vi "hw5_2_(2) - test.vi"() -> ()   [LabVIEW 2014]
panel:
  out "Display":string
  in  "stop":bool
  out "Result":string
  in  "Calculator":T1
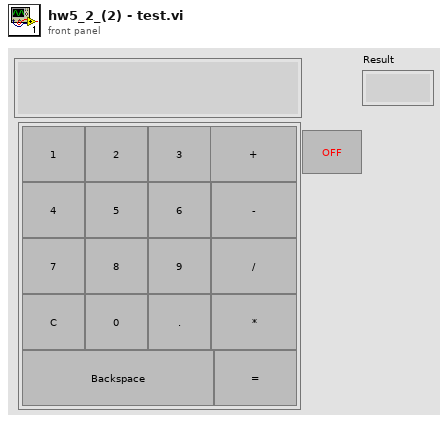
[diagram p1: front panel]
types:
  T1 = cluster{"2":bool, "3":bool, "4":bool, "5":bool, "6":bool, "7":bool, "8":bool, "9":bool, "*":bool, "=":bool, "backspace":bool, "0":bool, ".":bool, "C":bool, "/":bool, "-":bool, "+":bool, "1":bool}
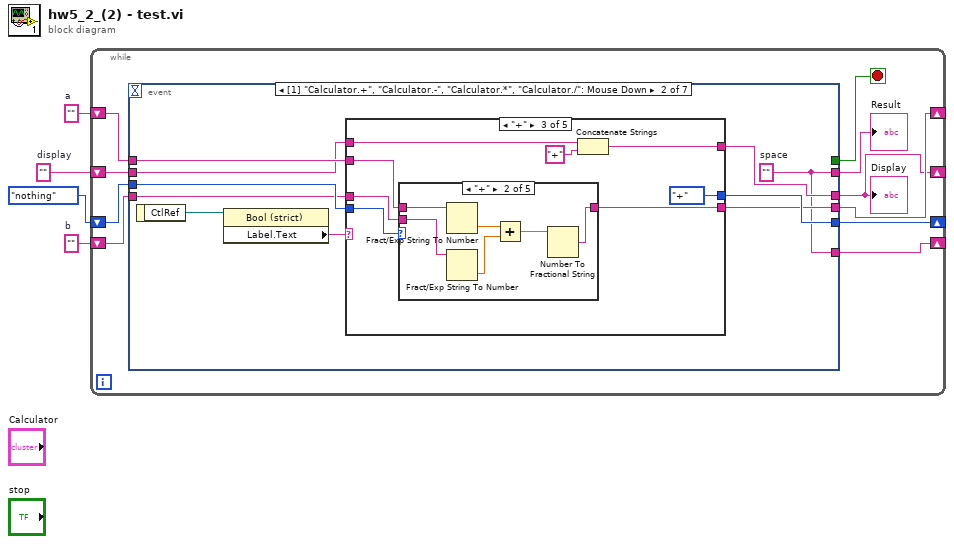
[diagram p0: block diagram]
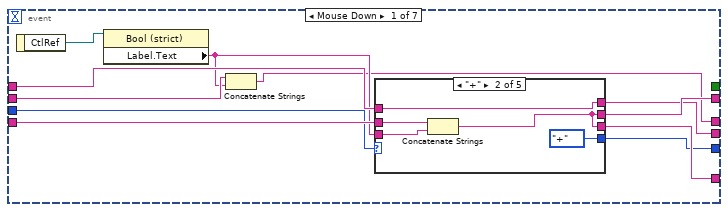
[diagram p2: hidden frame]
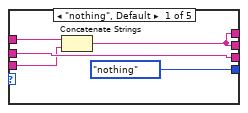
[diagram p3: hidden frame]
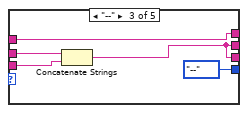
[diagram p4: hidden frame]
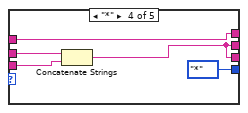
[diagram p5: hidden frame]
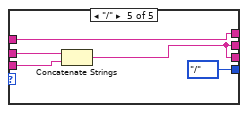
[diagram p6: hidden frame]
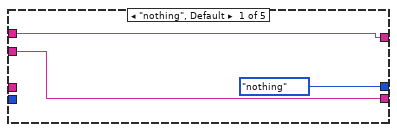
[diagram p7: hidden frame]
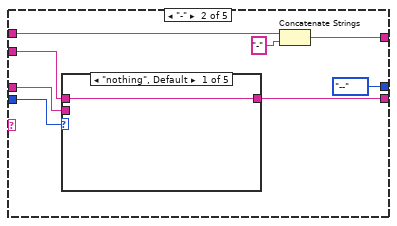
[diagram p8: hidden frame]
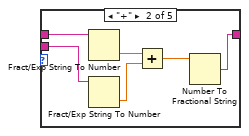
[diagram p9: hidden frame]
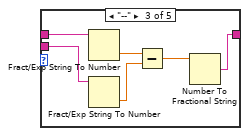
[diagram p10: hidden frame]
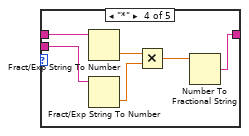
[diagram p11: hidden frame]
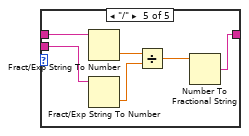
[diagram p12: hidden frame]
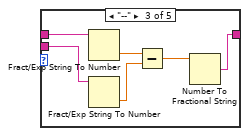
[diagram p14: hidden frame]
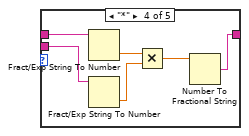
[diagram p15: hidden frame]
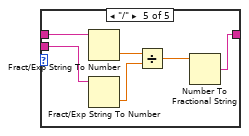
[diagram p16: hidden frame]
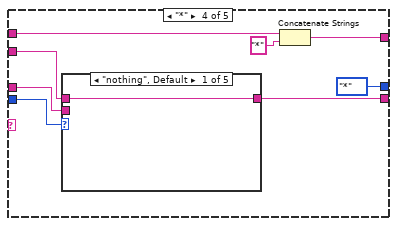
[diagram p17: hidden frame]
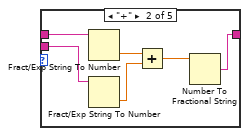
[diagram p18: hidden frame]
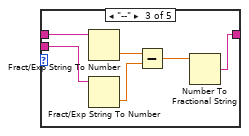
[diagram p19: hidden frame]
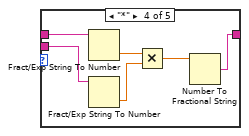
[diagram p20: hidden frame]
diagram:
  w1 = ""  # display
  w2 = ""  # b
  w4 = ""  # a
  n1 = while {
    shift-right: [w8] -> _
    shift-left: w4 -> [w14]
    shift-right: [w13] -> _
    shift-left: enum16{"nothing", "+", "--", "*", "/"}."nothing" -> [w10]
    shift-right: [w11] -> _
    shift-left: w2 -> [w12]
    shift-right: [w5] -> _
    shift-left: w1 -> [w6]
    stop <- w7 stop-if-true
    n2 = event shown="[1] \"Calculator.+\", \"Calculator.-\", \"Calculator.*\", \"Calculator./\": Mouse Down" {
      selector: _ -> [_ _ _ _ _ _ _]
      dyn-events: _ -> [_ _ _ _ _ _ _]
      timeout: _ -> [_ _ _ _ _ _ _]
      tunnel: w14 -> [w24 w58 w198 w241 w277 _ _]
      tunnel: [w18 w57 enum16{"nothing", "+", "--", "*", "/"}."nothing" w242 w281 _ _] -> w13
      tunnel: w12 -> [w23 w52 w197 w238 w276 _ _]
      tunnel: [w21 w51 w204 w243 w280 w312 _] -> w11
      tunnel: w10 -> [w19 w53 w199 w239 w275 _ _]
      tunnel: [w22 w51 w196 w244 w279 w312 _] -> w9
      tunnel: [w20 w56 w196 w245 w278 w312 _] -> w8
      tunnel: [_ _ _ _ _ _ TRUE] -> w7
      tunnel: w6 -> [w17 w54 w203 w237 w272 _ _]
      tunnel: [w15 w55 w200 w235 w271 w312 _] -> w5
      event "Calculator.1", "Calculator.2", "Calculator.3", "Calculator.4", "Calculator.5", "Calculator.6", "Calculator.7", "Calculator.8", "Calculator.9", "Calculator.0": Mouse Down {
        n3 = event-data() -> ("CtlRef"=w25:refnum<vi>)  [unwired: 1 in]
        n4 = property class="Bool (strict)"(reference=w25) -> ("Label.Text"=w16:string)  [unwired: 1 in, 2 out]
        n5 = Concatenate Strings(w17, w16) -> (w15:string)
        n6 = case shown="\"+\"" w19 {
          tunnel: w24 -> [w29 w34 w39 w44 w49]
          tunnel: w16 -> [w26 w31 w36 w41 w46]
          tunnel: [w27 w32 w37 w42 w48] -> w22
          tunnel: w23 -> [w30 w35 w40 w45 w50]
          tunnel: [w30 w32 w37 w42 w48] -> w21
          tunnel: [w27 w34 w39 w44 w49] -> w20
          tunnel: [enum16{"nothing", "+", "--", "*", "/"}."nothing" enum16{"nothing", "+", "--", "*", "/"}."+" enum16{"nothing", "+", "--", "*", "/"}."--" enum16{"nothing", "+", "--", "*", "/"}."*" enum16{"nothing", "+", "--", "*", "/"}."/"] -> w18
          frame "nothing", Default {
            n7 = Concatenate Strings(w29, w26) -> (w27:string)
          }
          frame "+" {
            n8 = Concatenate Strings(w35, w31) -> (w32:string)
          }
          frame "--" {
            n9 = Concatenate Strings(w40, w36) -> (w37:string)
          }
          frame "*" {
            n10 = Concatenate Strings(w45, w41) -> (w42:string)
          }
          frame "/" {
            n11 = Concatenate Strings(w50, w46) -> (w48:string)
          }
        }
      }
      event "Calculator.+", "Calculator.-", "Calculator.*", "Calculator./": Mouse Down {
        w51 = ""  # space
        n12 = event-data() -> ("CtlRef"=w60:refnum<vi>)  [unwired: 1 in]
        n13 = property class="Bool (strict)"(reference=w60) -> ("Label.Text"=w59:string)  [unwired: 1 in, 2 out]
        n14 = case shown="\"+\"" w59 {
          tunnel: w52 -> [_ w65 w98 w131 w164]
          tunnel: [w63 w67 w100 w133 w166] -> w56
          tunnel: w58 -> [w63 w71 w104 w137 w170]
          tunnel: [enum16{"nothing", "+", "--", "*", "/"}."nothing" enum16{"nothing", "+", "--", "*", "/"}."--" enum16{"nothing", "+", "--", "*", "/"}."+" enum16{"nothing", "+", "--", "*", "/"}."*" enum16{"nothing", "+", "--", "*", "/"}."/"] -> w57
          tunnel: [w61 w69 w102 w135 w168] -> w55
          tunnel: w54 -> [w61 w66 w99 w132 w165]
          tunnel: w53 -> [_ w64 w97 w130 w163]
          frame "nothing", Default {
          }
          frame "-" {
            n15 = case shown="\"nothing\", Default" w64 {
              tunnel: w71 -> [w72 w78 w84 w90 w96]
              tunnel: [w72 w77 w83 w89 w95] -> w67
              tunnel: w65 -> [_ w74 w80 w86 w92]
              frame "nothing", Default {
              }
              frame "+" {
                n16 = Fract/Exp String To Number(string=w78) -> (number=w75:dbl)  [unwired: 3 in, 1 out]
                n17 = Fract/Exp String To Number(string=w74) -> (number=w76:dbl)  [unwired: 3 in, 1 out]
                n18 = Add(x=w75, y=w76) -> (x+y=w73:dbl)
                n19 = Number To Fractional String(number=w73) -> (F-format string=w77:string)  [unwired: 3 in]
              }
              frame "--" {
                n20 = Fract/Exp String To Number(string=w84) -> (number=w81:dbl)  [unwired: 3 in, 1 out]
                n21 = Fract/Exp String To Number(string=w80) -> (number=w82:dbl)  [unwired: 3 in, 1 out]
                n22 = Subtract(x=w81, y=w82) -> (x-y=w79:dbl)
                n23 = Number To Fractional String(number=w79) -> (F-format string=w83:string)  [unwired: 3 in]
              }
              frame "*" {
                n24 = Fract/Exp String To Number(string=w90) -> (number=w87:dbl)  [unwired: 3 in, 1 out]
                n25 = Fract/Exp String To Number(string=w86) -> (number=w88:dbl)  [unwired: 3 in, 1 out]
                n26 = Multiply(x=w87, y=w88) -> (x*y=w85:dbl)
                n27 = Number To Fractional String(number=w85) -> (F-format string=w89:string)  [unwired: 3 in]
              }
              frame "/" {
                n28 = Fract/Exp String To Number(string=w96) -> (number=w93:dbl)  [unwired: 3 in, 1 out]
                n29 = Fract/Exp String To Number(string=w92) -> (number=w94:dbl)  [unwired: 3 in, 1 out]
                n30 = Divide(x=w93, y=w94) -> (x/y=w91:dbl)
                n31 = Number To Fractional String(number=w91) -> (F-format string=w95:string)  [unwired: 3 in]
              }
            }
            n32 = Concatenate Strings(w66, "-") -> (w69:string)
          }
          frame "+" {
            n33 = case shown="\"+\"" w97 {
              tunnel: w104 -> [w105 w111 w117 w123 w129]
              tunnel: [w105 w110 w116 w122 w128] -> w100
              tunnel: w98 -> [_ w107 w113 w119 w125]
              frame "nothing", Default {
              }
              frame "+" {
                n34 = Fract/Exp String To Number(string=w111) -> (number=w108:dbl)  [unwired: 3 in, 1 out]
                n35 = Fract/Exp String To Number(string=w107) -> (number=w109:dbl)  [unwired: 3 in, 1 out]
                n36 = Add(x=w108, y=w109) -> (x+y=w106:dbl)
                n37 = Number To Fractional String(number=w106) -> (F-format string=w110:string)  [unwired: 3 in]
              }
              frame "--" {
                n38 = Fract/Exp String To Number(string=w117) -> (number=w114:dbl)  [unwired: 3 in, 1 out]
                n39 = Fract/Exp String To Number(string=w113) -> (number=w115:dbl)  [unwired: 3 in, 1 out]
                n40 = Subtract(x=w114, y=w115) -> (x-y=w112:dbl)
                n41 = Number To Fractional String(number=w112) -> (F-format string=w116:string)  [unwired: 3 in]
              }
              frame "*" {
                n42 = Fract/Exp String To Number(string=w123) -> (number=w120:dbl)  [unwired: 3 in, 1 out]
                n43 = Fract/Exp String To Number(string=w119) -> (number=w121:dbl)  [unwired: 3 in, 1 out]
                n44 = Multiply(x=w120, y=w121) -> (x*y=w118:dbl)
                n45 = Number To Fractional String(number=w118) -> (F-format string=w122:string)  [unwired: 3 in]
              }
              frame "/" {
                n46 = Fract/Exp String To Number(string=w129) -> (number=w126:dbl)  [unwired: 3 in, 1 out]
                n47 = Fract/Exp String To Number(string=w125) -> (number=w127:dbl)  [unwired: 3 in, 1 out]
                n48 = Divide(x=w126, y=w127) -> (x/y=w124:dbl)
                n49 = Number To Fractional String(number=w124) -> (F-format string=w128:string)  [unwired: 3 in]
              }
            }
            n50 = Concatenate Strings(w99, "+") -> (w102:string)
          }
          frame "*" {
            n51 = case shown="\"nothing\", Default" w130 {
              tunnel: w137 -> [w138 w144 w150 w156 w162]
              tunnel: [w138 w143 w149 w155 w161] -> w133
              tunnel: w131 -> [_ w140 w146 w152 w158]
              frame "nothing", Default {
              }
              frame "+" {
                n52 = Fract/Exp String To Number(string=w144) -> (number=w141:dbl)  [unwired: 3 in, 1 out]
                n53 = Fract/Exp String To Number(string=w140) -> (number=w142:dbl)  [unwired: 3 in, 1 out]
                n54 = Add(x=w141, y=w142) -> (x+y=w139:dbl)
                n55 = Number To Fractional String(number=w139) -> (F-format string=w143:string)  [unwired: 3 in]
              }
              frame "--" {
                n56 = Fract/Exp String To Number(string=w150) -> (number=w147:dbl)  [unwired: 3 in, 1 out]
                n57 = Fract/Exp String To Number(string=w146) -> (number=w148:dbl)  [unwired: 3 in, 1 out]
                n58 = Subtract(x=w147, y=w148) -> (x-y=w145:dbl)
                n59 = Number To Fractional String(number=w145) -> (F-format string=w149:string)  [unwired: 3 in]
              }
              frame "*" {
                n60 = Fract/Exp String To Number(string=w156) -> (number=w153:dbl)  [unwired: 3 in, 1 out]
                n61 = Fract/Exp String To Number(string=w152) -> (number=w154:dbl)  [unwired: 3 in, 1 out]
                n62 = Multiply(x=w153, y=w154) -> (x*y=w151:dbl)
                n63 = Number To Fractional String(number=w151) -> (F-format string=w155:string)  [unwired: 3 in]
              }
              frame "/" {
                n64 = Fract/Exp String To Number(string=w162) -> (number=w159:dbl)  [unwired: 3 in, 1 out]
                n65 = Fract/Exp String To Number(string=w158) -> (number=w160:dbl)  [unwired: 3 in, 1 out]
                n66 = Divide(x=w159, y=w160) -> (x/y=w157:dbl)
                n67 = Number To Fractional String(number=w157) -> (F-format string=w161:string)  [unwired: 3 in]
              }
            }
            n68 = Concatenate Strings(w132, "*") -> (w135:string)
          }
          frame "/" {
            n69 = case shown="\"nothing\", Default" w163 {
              tunnel: w170 -> [w171 w177 w183 w189 w195]
              tunnel: [w171 w176 w182 w188 w194] -> w166
              tunnel: w164 -> [_ w173 w179 w185 w191]
              frame "nothing", Default {
              }
              frame "+" {
                n70 = Fract/Exp String To Number(string=w177) -> (number=w174:dbl)  [unwired: 3 in, 1 out]
                n71 = Fract/Exp String To Number(string=w173) -> (number=w175:dbl)  [unwired: 3 in, 1 out]
                n72 = Add(x=w174, y=w175) -> (x+y=w172:dbl)
                n73 = Number To Fractional String(number=w172) -> (F-format string=w176:string)  [unwired: 3 in]
              }
              frame "--" {
                n74 = Fract/Exp String To Number(string=w183) -> (number=w180:dbl)  [unwired: 3 in, 1 out]
                n75 = Fract/Exp String To Number(string=w179) -> (number=w181:dbl)  [unwired: 3 in, 1 out]
                n76 = Subtract(x=w180, y=w181) -> (x-y=w178:dbl)
                n77 = Number To Fractional String(number=w178) -> (F-format string=w182:string)  [unwired: 3 in]
              }
              frame "*" {
                n78 = Fract/Exp String To Number(string=w189) -> (number=w186:dbl)  [unwired: 3 in, 1 out]
                n79 = Fract/Exp String To Number(string=w185) -> (number=w187:dbl)  [unwired: 3 in, 1 out]
                n80 = Multiply(x=w186, y=w187) -> (x*y=w184:dbl)
                n81 = Number To Fractional String(number=w184) -> (F-format string=w188:string)  [unwired: 3 in]
              }
              frame "/" {
                n82 = Fract/Exp String To Number(string=w195) -> (number=w192:dbl)  [unwired: 3 in, 1 out]
                n83 = Fract/Exp String To Number(string=w191) -> (number=w193:dbl)  [unwired: 3 in, 1 out]
                n84 = Divide(x=w192, y=w193) -> (x/y=w190:dbl)
                n85 = Number To Fractional String(number=w190) -> (F-format string=w194:string)  [unwired: 3 in]
              }
            }
            n86 = Concatenate Strings(w165, "/") -> (w168:string)
          }
        }
      }
      event "Calculator.=": Mouse Down {
        w204 = ""  # b
        n87 = event-data() -> ()  [unwired: 1 in, 1 out]
        n88 = case shown="\"nothing\", Default" w199 {
          tunnel: w197 -> [_ w210 w217 w224 w232]
          tunnel: [w206 w209 w216 w223 w230] -> w196
          tunnel: w198 -> [w206 w208 w215 w222 w229]
          tunnel: [enum16{"nothing", "+", "--", "*", "/"}."nothing" enum16{"nothing", "+", "--", "*", "/"}."+" enum16{"nothing", "+", "--", "*", "/"}."--" enum16{"nothing", "+", "--", "*", "/"}."*" enum16{"nothing", "+", "--", "*", "/"}."/"] -> _
          frame "nothing", Default {
          }
          frame "+" {
            n89 = Fract/Exp String To Number(string=w208) -> (number=w213:dbl)  [unwired: 3 in, 1 out]
            n90 = Fract/Exp String To Number(string=w210) -> (number=w212:dbl)  [unwired: 3 in, 1 out]
            n91 = Add(x=w213, y=w212) -> (x+y=w211:dbl)
            n92 = Number To Fractional String(number=w211) -> (F-format string=w209:string)  [unwired: 3 in]
          }
          frame "--" {
            n93 = Fract/Exp String To Number(string=w215) -> (number=w220:dbl)  [unwired: 3 in, 1 out]
            n94 = Fract/Exp String To Number(string=w217) -> (number=w219:dbl)  [unwired: 3 in, 1 out]
            n95 = Subtract(x=w220, y=w219) -> (x-y=w218:dbl)
            n96 = Number To Fractional String(number=w218) -> (F-format string=w216:string)  [unwired: 3 in]
          }
          frame "*" {
            n97 = Fract/Exp String To Number(string=w222) -> (number=w227:dbl)  [unwired: 3 in, 1 out]
            n98 = Fract/Exp String To Number(string=w224) -> (number=w226:dbl)  [unwired: 3 in, 1 out]
            n99 = Multiply(x=w227, y=w226) -> (x*y=w225:dbl)
            n100 = Number To Fractional String(number=w225) -> (F-format string=w223:string)  [unwired: 3 in]
          }
          frame "/" {
            n101 = Fract/Exp String To Number(string=w229) -> (number=w234:dbl)  [unwired: 3 in, 1 out]
            n102 = Fract/Exp String To Number(string=w232) -> (number=w233:dbl)  [unwired: 3 in, 1 out]
            n103 = Divide(x=w234, y=w233) -> (x/y=w231:dbl)
            n104 = Number To Fractional String(number=w231) -> (F-format string=w230:string)  [unwired: 3 in]
          }
        }
        n105 = Concatenate Strings(w203, "=" ("string"), w196) -> (w200:string)
      }
      event "Calculator..": Mouse Down {
        n106 = event-data() -> ("CtlRef"=w240:refnum<vi>)  [unwired: 1 in]
        n107 = property class="Bool (strict)"(reference=w240) -> ("Label.Text"=w236:string)  [unwired: 1 in, 2 out]
        n108 = Concatenate Strings(w237, w236) -> (w235:string)
        n109 = case shown="\"nothing\", Default" w239 {
          tunnel: w241 -> [w249 w254 w259 w264 w269]
          tunnel: w236 -> [w246 w251 w256 w261 w266]
          tunnel: [w248 w253 w258 w263 w268] -> w244
          tunnel: w238 -> [w250 w255 w260 w265 w270]
          tunnel: [w250 w253 w258 w263 w268] -> w243
          tunnel: [w248 w254 w259 w264 w269] -> w245
          tunnel: [enum16{"nothing", "+", "--", "*", "/"}."nothing" enum16{"nothing", "+", "--", "*", "/"}."+" enum16{"nothing", "+", "--", "*", "/"}."--" enum16{"nothing", "+", "--", "*", "/"}."*" enum16{"nothing", "+", "--", "*", "/"}."/"] -> w242
          frame "nothing", Default {
            n110 = Concatenate Strings(w249, w246) -> (w248:string)
          }
          frame "+" {
            n111 = Concatenate Strings(w255, w251) -> (w253:string)
          }
          frame "--" {
            n112 = Concatenate Strings(w260, w256) -> (w258:string)
          }
          frame "*" {
            n113 = Concatenate Strings(w265, w261) -> (w263:string)
          }
          frame "/" {
            n114 = Concatenate Strings(w270, w266) -> (w268:string)
          }
        }
      }
      event "Calculator.backspace": Mouse Down {
        n115 = event-data() -> ()  [unwired: 1 in, 1 out]
        n116 = String Length(string=w272) -> (length=w274:i32)
        n117 = Decrement(x=w274) -> (x-1=w273:i32)
        n118 = String Subset(string=w272, length (rest)=w273) -> (substring=w271:string)  [unwired: 1 in]
        n119 = case shown="\"nothing\", Default" w275 {
          tunnel: w277 -> [w284 w291 w297 w303 w309]
          tunnel: [w286 w289 w295 w301 w307] -> w279
          tunnel: w276 -> [w287 w290 w296 w302 w308]
          tunnel: [w287 w289 w295 w301 w307] -> w280
          tunnel: [w286 w291 w297 w303 w309] -> w278
          tunnel: [enum16{"nothing", "+", "--", "*", "/"}."nothing" enum16{"nothing", "+", "--", "*", "/"}."+" enum16{"nothing", "+", "--", "*", "/"}."--" enum16{"nothing", "+", "--", "*", "/"}."*" enum16{"nothing", "+", "--", "*", "/"}."/"] -> w281
          frame "nothing", Default {
            n120 = String Length(string=w284) -> (length=w283:i32)
            n121 = Decrement(x=w283) -> (x-1=w282:i32)
            n122 = String Subset(string=w284, length (rest)=w282) -> (substring=w286:string)  [unwired: 1 in]
          }
          frame "+" {
            n123 = String Length(string=w290) -> (length=w292:i32)
            n124 = Decrement(x=w292) -> (x-1=w288:i32)
            n125 = String Subset(string=w290, length (rest)=w288) -> (substring=w289:string)  [unwired: 1 in]
          }
          frame "--" {
            n126 = String Length(string=w296) -> (length=w298:i32)
            n127 = Decrement(x=w298) -> (x-1=w294:i32)
            n128 = String Subset(string=w296, length (rest)=w294) -> (substring=w295:string)  [unwired: 1 in]
          }
          frame "*" {
            n129 = String Length(string=w302) -> (length=w304:i32)
            n130 = Decrement(x=w304) -> (x-1=w300:i32)
            n131 = String Subset(string=w302, length (rest)=w300) -> (substring=w301:string)  [unwired: 1 in]
          }
          frame "/" {
            n132 = String Length(string=w308) -> (length=w310:i32)
            n133 = Decrement(x=w310) -> (x-1=w306:i32)
            n134 = String Subset(string=w308, length (rest)=w306) -> (substring=w307:string)  [unwired: 1 in]
          }
        }
      }
      event "Calculator.C": Mouse Down {
        w312 = ""  # null
        n135 = event-data() -> ()  [unwired: 1 in, 8 out]
      }
      event "stop": Mouse Down {
        n136 = event-data() -> ()  [unwired: 1 in, 8 out]
      }
    }
    "Result" <- w9
    "Display" <- w5
  }
